vi "main.vi"() -> ()   [LabVIEW 2019]
uses:
  Type defs/Loop data Type Def.ctl
  Type defs/Persistent Type Def.ctl
  Type defs/Temp handle Type Def.ctl
  Type defs/Temp ctrl Type Def.ctl
  Custom devices/Custom temp ctrl settings.ctl
  Type defs/Paths Type Def.ctl
  Type defs/Settings Type Def.ctl
  Type defs/Imps Type Def.ctl
  Type defs/Source-meter Type Def.ctl
  Custom devices/Custom source-meter settings.ctl
  Type defs/Other settings Type Def.ctl
  Type defs/IV properties Type Def.ctl
  Type defs/CV properties Type Def.ctl
  Type defs/DLTS properties Type Def.ctl
  Type defs/LDLTS properties Type Def.ctl
  Type defs/MFIA handle Type Def.ctl
  <instrlib>/Zurich Instruments LabOne/Public/ziTypeHandle.ctl
  <instrlib>/Zurich Instruments LabOne/Public/Modules/ziTypeModHandle.ctl
  Type defs/Source-meter handle Type Def.ctl
  <vilib>/Utility/sysdir.llb/System Directory Type.ctl
  <vilib>/Utility/miscctls.llb/LVPointTypeDef.ctl
  <vilib>/Utility/error.llb/DialogType.ctl
  <instrlib>/Zurich Instruments LabOne/Zurich Instruments LabOne.lvlib
panel:
  out "Version":dbl caption="Numeric" format="myDLTS %.;%.2g"
  in  "Help":bool
  in  "Settings":bool
  in  "Path":path
  in  "File Open":bool
  in  "Add":bool
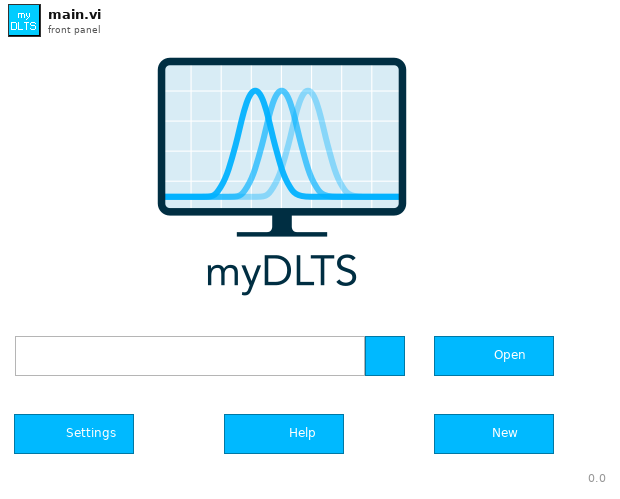
[diagram p1: front panel]
types:
  T1 = enum32{"Invalid", "Standard", "Closed", "Hidden", "Minimized", "Maximized"}
  T2 = typedef "System Directory Type.ctl" = i32
  T3 = typedef "LVPointTypeDef.ctl" = cluster{"Horizontal":i16, "Vertical":i16}
  T4 = typedef "Loop data Type Def.ctl" = cluster{"Persistent":T5, "Temp handle":T6, "Paths":T9, "Settings":T10, "Software version":dbl, "MFIA handle":T19, "Source-meter handle":T22}
  T5 = typedef "Persistent Type Def.ctl" = cluster{"Last file":path, "Last user":string, "Users":cluster{"User":string, "Authors directory":path}[]}
  T6 = typedef "Temp handle Type Def.ctl" = cluster{"Connected":bool, "Temp ctrl":T7}
  T7 = typedef "Temp ctrl Type Def.ctl" = cluster{"Gain (P)":dbl, "Reset (I)":dbl, "Rate (D)":dbl, "Stabilization rate":dbl, "Stabilization delta":dbl, "Type":enum16{"Custom", "Lake Shore 325", "Lake Shore 331", "Lake Shore 332", "Lake Shore 335"}, "Custom temp ctrl":T8, "Lakeshore 325":cluster{"VISA name":refnum<visa-resource-name>, "Loop":u16, "Heater Range":u16, "Heater Resistance":u16, "Sample sensor":u16, "Fast sensor":u16, "Slow sensor":u16}, "Lakeshore 331":cluster{"VISA name":refnum<visa-resource-name>, "Loop":u16, "Heater Range":u16, "Sample sensor":u16, "Fast sensor":u16, "Slow sensor":u16}, "Lakeshore 332":cluster{"VISA name":refnum<visa-resource-name>, "Loop":u16, "Heater Range":u16, "Sample sensor":u16, "Fast sensor":u16, "Slow sensor":u16}, "Lakeshore 335":cluster{"VISA name":refnum<visa-resource-name>, "Loop":u16, "Sample sensor":u16, "Fast sensor":u16, "Slow sensor":u16, "Heater Range":u16, "Output mode":enum16{"Off", "Closed Loop PID", "Zone", "Open Loop", "Monitor Out", "Warmup Supply"}}}
  T8 = typedef "Custom temp ctrl settings.ctl" = cluster{"VISA resource name":refnum<visa-resource-name>}
  T9 = typedef "Paths Type Def.ctl" = cluster{"Manual":path, "Settings":path, "Persistent":path, "Work dir.":path}
  T10 = typedef "Settings Type Def.ctl" = cluster{"MFIA":T11, "Temp ctrl":T7, "Source-meter":T12, "Other":T14, "Defaults":cluster{"IV properties":T15, "CV properties":T16, "DLTS properties":T17, "LDLTS properties":T18}}
  T11 = typedef "Imps Type Def.ctl" = cluster{"Address":string, "Use compensation":bool, "Shut down gracefully":bool}
  T12 = typedef "Source-meter Type Def.ctl" = cluster{"Type":enum16{"Custom", "Keithley 2600"}, "Custom source-meter":T13, "Keithley 2600":cluster{"VISA name":refnum<visa-resource-name>}}
  T13 = typedef "Custom source-meter settings.ctl" = cluster{"VISA resource name":refnum<visa-resource-name>}
  T14 = typedef "Other settings Type Def.ctl" = cluster{"Enable OriginLab":bool, "Reader mode":bool, "Auto-save":bool}
  T15 = typedef "IV properties Type Def.ctl" = cluster{"T":dbl[unit], "Vstart":dbl[unit], "Vstop":dbl[unit], "Vpoints":dbl, "Settling":dbl[unit], "I limit":dbl[unit], "Log mapping":bool, "Averaging":dbl}
  T16 = typedef "CV properties Type Def.ctl" = cluster{"T":dbl[unit], "Vstart":dbl[unit], "Vstop":dbl[unit], "Vpoints":dbl, "Precision":enum16{"Low (Fast)", "Normal", "High (Slow)"}, "Test signal":dbl[unit], "Auto I range":bool, "Test frequency":dbl[unit], "I range":dbl, "V range":dbl[unit], "Log mapping":bool, "Rel perm":dbl, "Area":dbl[unit]}
  T17 = typedef "DLTS properties Type Def.ctl" = cluster{"Tstart":dbl[unit], "Instant start":bool, "Tstop":dbl[unit], "T rate":dbl[unit], "Test signal":dbl[unit], "Test frequency":dbl[unit], "Bandwidth":dbl[unit], "Averaging":dbl, "Vbias":dbl[unit], "Vpulse":dbl[unit], "pulse length":dbl[unit], "Pulse 2":bool, "Vpulse 2":dbl[unit], "pulse length 2":dbl[unit], "I range":dbl, "V range":dbl[unit], "Emission rate":dbl[unit][], "Sampling rate":dbl[unit], "Acq. delay":dbl[unit]}
  T18 = typedef "LDLTS properties Type Def.ctl" = cluster{"T":dbl[unit], "Test signal":dbl[unit], "Test frequency":dbl[unit], "Bandwidth":dbl[unit], "Averaging":dbl, "Vbias":dbl[unit], "Vpulse":dbl[unit], "pulse length":dbl[unit], "Pulse 2":bool, "Vpulse 2":dbl[unit], "pulse length 2":dbl[unit], "I range":dbl, "V range":dbl[unit], "Sampling rate":dbl[unit], "Acq. delay":dbl[unit], "Sampling time":dbl[unit]}
  T19 = typedef "MFIA handle Type Def.ctl" = cluster{"ziHandle":T20, "Selected device":string, "ziModHandle":T21}
  T20 = typedef "Zurich Instruments LabOne.lvlib/ziTypeHandle.ctl" = cluster{"handleValid":bool, "Conn":u64, "Path Prefix":string, "Handle":u64, "Connected":bool, "Clockbase(s)":dbl}
  T21 = typedef "Zurich Instruments LabOne.lvlib/ziTypeModHandle.ctl" = cluster{"handleValid":bool, "Conn":u64, "ModHandle":u64, "moduleID":string, "Path Prefix":string}
  T22 = typedef "Source-meter handle Type Def.ctl" = cluster{"Connected":bool, "Source-meter":T12}
  T23 = enum8{"Enabled", "Disabled", "Disabled and Grayed Out"}
  T24 = typedef "DialogType.ctl" = u16
  T25 = typedef "Session properties Type Def.ctl" = cluster{"Session name":string, "Comment":string, "User":string, "Software version":dbl, "Created":timestamp, "Modified":timestamp, "Binary":bool, "GUID":string}
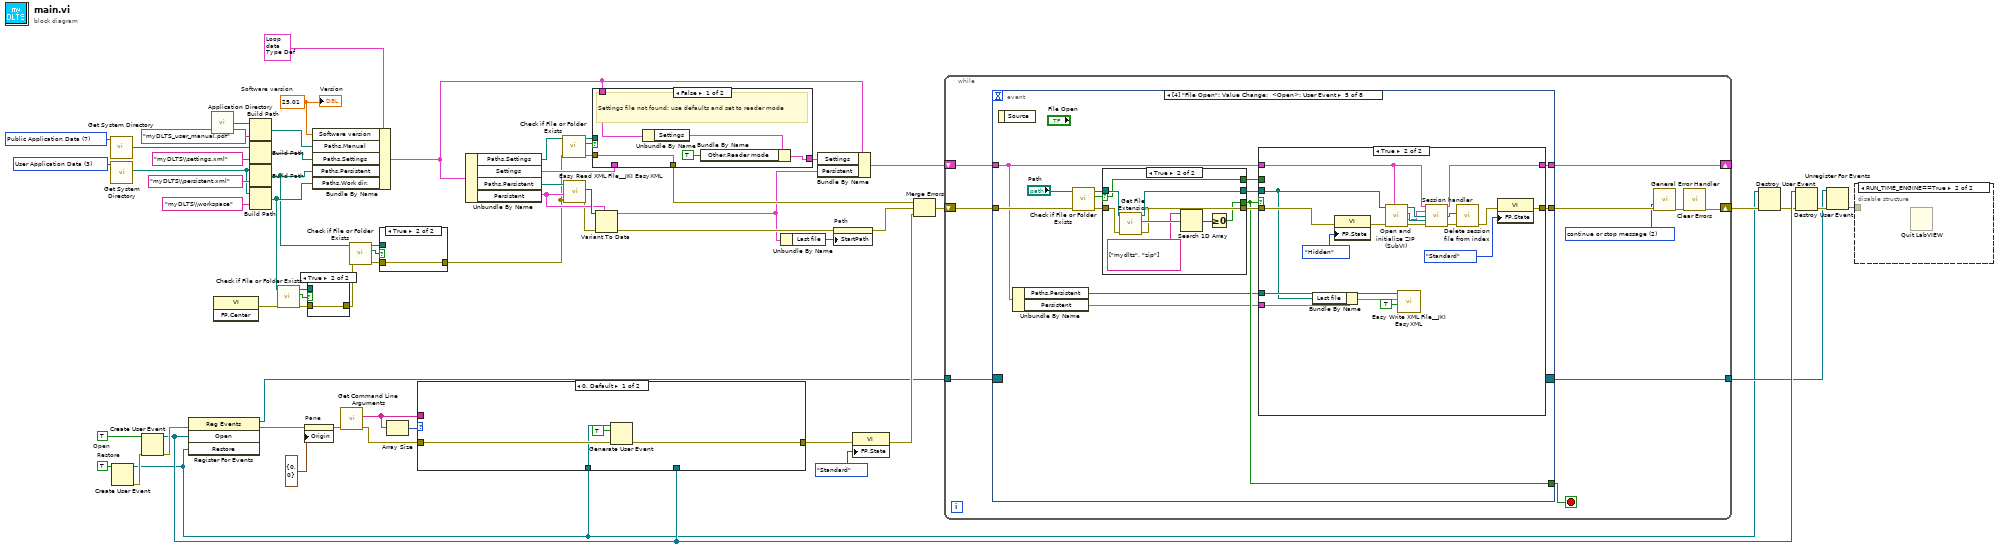
[diagram p0: block diagram]
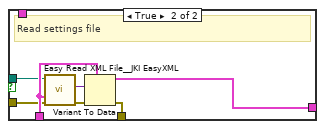
[diagram p2: hidden frame]
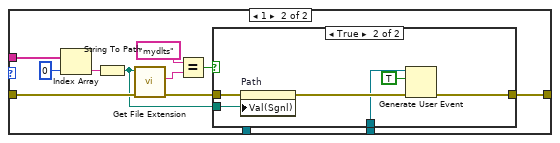
[diagram p4: hidden frame]
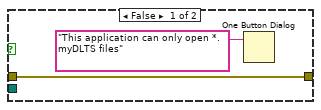
[diagram p5: hidden frame]
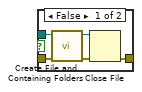
[diagram p6: hidden frame]
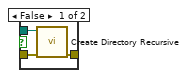
[diagram p7: hidden frame]
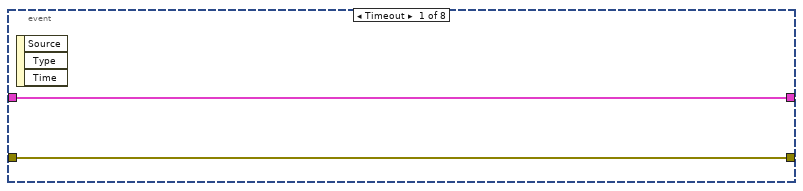
[diagram p8: hidden frame]
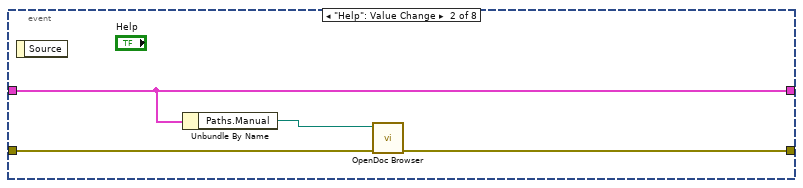
[diagram p9: hidden frame]
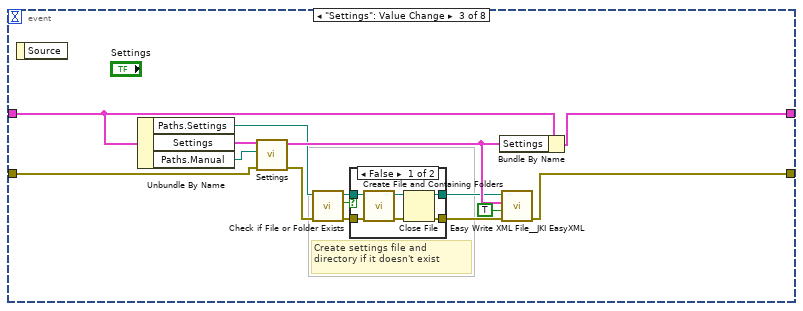
[diagram p10: hidden frame]
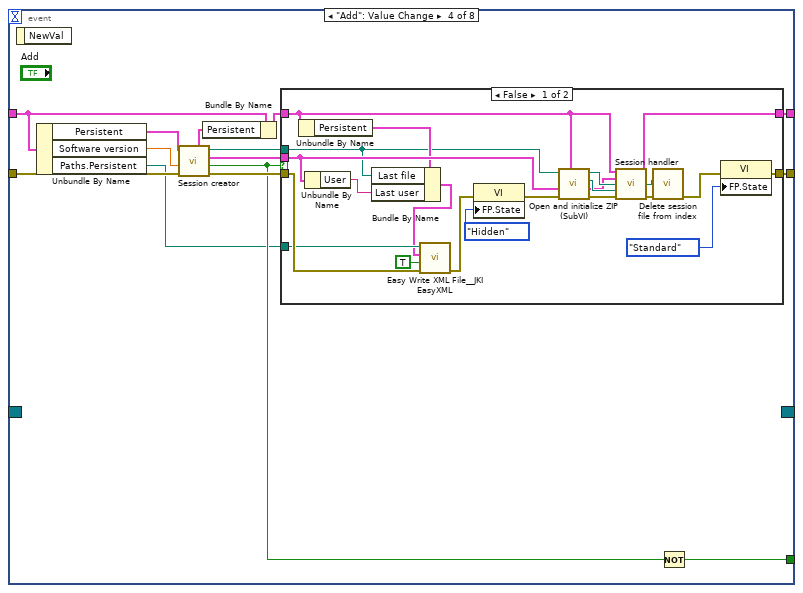
[diagram p12: hidden frame]
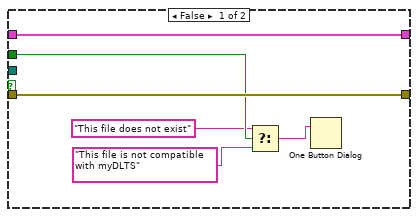
[diagram p15: hidden frame]
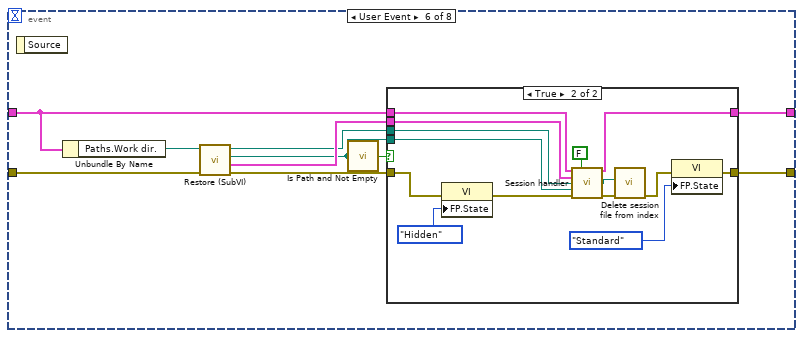
[diagram p16: hidden frame]
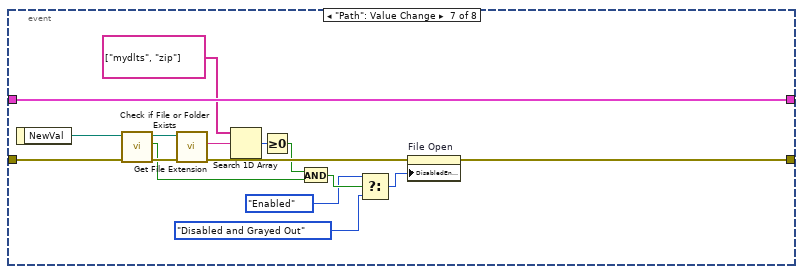
[diagram p18: hidden frame]
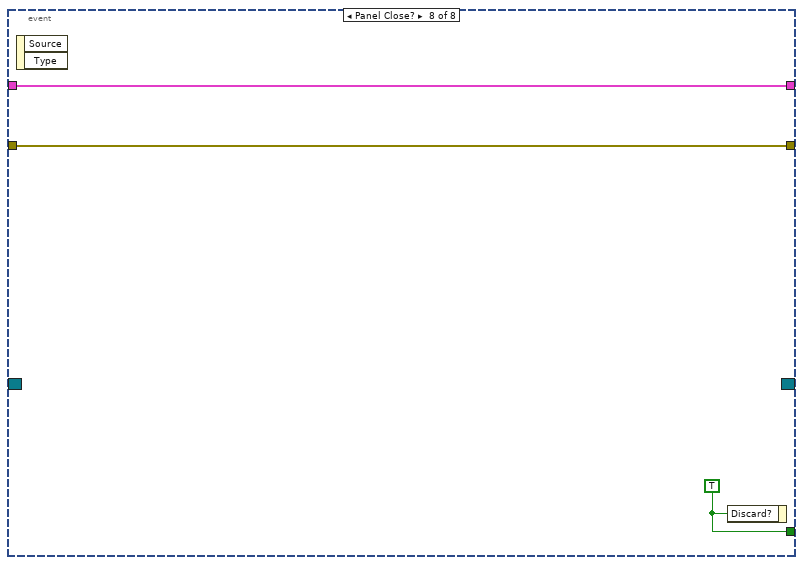
[diagram p19: hidden frame]
diagram:
  w1 = 25.01  # Software version
  w12 = TRUE  # Restore
  w20 = TRUE  # Open
  w30 = T2 7 items=["User Home"=0, "User Desktop"=1, "User Documents"=2, "User Application Data"=3, "User Preferences"=4, "User Temporary"=5, "Public Documents"=6, "Public Application Data"=7, "Public Preferences"=8, "Public Cache"=13, "System Core Libraries"=9, "System Installed Libraries"=10, "Application Files"=11, "Boot Volume Root"=12] ("system directory type")
  w59 = T2 3 items=["User Home"=0, "User Desktop"=1, "User Documents"=2, "User Application Data"=3, "User Preferences"=4, "User Temporary"=5, "Public Documents"=6, "Public Application Data"=7, "Public Preferences"=8, "Public Cache"=13, "System Core Libraries"=9, "System Installed Libraries"=10, "Application Files"=11, "Boot Volume Root"=12] ("system directory type")
  n1 = call <vilib>:"Get System Directory.vi"("system directory type"=w30) -> ("system directory"=w29:path)  [unwired: 10 in]
  n2 = call <vilib>:"Get System Directory.vi"("system directory type"=w59) -> ("system directory"=w56:path)  [unwired: 10 in]
  n3 = Create User Event(user event datatype=w12) -> (user event=w8:refnum<user-event>, error out=w11:errorcluster)  [unwired: 1 in]
  n4 = Create User Event(user event datatype=w20, error in=w11) -> (user event=w16:refnum<user-event>, error out=w17:errorcluster)
  n5 = register-events(error in=w17, w16, w8) -> (reference out=w18:refnum<event-registration>, error out=w19:errorcluster)  [unwired: 1 in]
  n6 = call <vilib>:"Application Directory.vi"() -> ("Application Directory"=w62:path)
  n7 = invoke class="VI" method="FP.Center"() -> (error out=w21:errorcluster)  [unwired: 3 in, 2 out]
  n8 = Build Path(base path=w62, name or relative path="myDLTS_user_manual.pdf") -> (appended path=w60:path)
  n9 = Build Path(base path=w29, name or relative path="myDLTS\\settings.xml") -> (appended path=w36:path)
  n10 = Build Path(base path=w56, name or relative path="myDLTS\\persistent.xml") -> (appended path=w38:path)
  n11 = Build Path(base path=w56, name or relative path="myDLTS\\workspace") -> (appended path=w45:path)
  n12 = call <vilib>:"Check if File or Folder Exists.vi"("error in (no error)"=w21, "path"=w45) -> ("error out"=w43:errorcluster, "file or folder exists?"=w42:bool, "dup path"=w44:path)  [unwired: 7 in]
  n13 = property on="Pane" class="Pane"(error in=w19, "Origin"=T3 {"Horizontal"=0, "Vertical"=0}) -> (error out=w32:errorcluster)  [unwired: 1 in, 1 out]
  n14 = case shown="True" w42 {
    tunnel: w44 -> [w66 _]
    tunnel: w43 -> [w65 w67]
    tunnel: [w64 w67] -> w37
    frame False {
      n15 = call <vilib>:"Create Directory Recursive.vi"("error in (no error)"=w65, "directory"=w66) -> ("error out"=w64:errorcluster)  [unwired: 3 in, 2 out]
    }
    frame True {
    }
  }
  n16 = Bundle By Name(cluster=T4 {"Persistent"={"Last file"=path "", "Last user"="", "Users"=[]}, "Temp handle"={"Connected"=FALSE, "Temp ctrl"={"Gain (P)"=0.0, "Reset (I)"=0.0, "Rate (D)"=0.0, "Stabilization rate"=0.0, "Stabilization delta"=0.0, "Type"=enum."Lake Shore 325", "Custom temp ctrl"={"VISA resource name"=""}, "Lakeshore 325"={"VISA name"="", "Loop"=0, "Heater Range"=1, "Heater Resistance"=0, "Sample sensor"=0, "Fast sensor"=0, "Slow sensor"=0}, "Lakeshore 331"={"VISA name"="", "Loop"=1, "Heater Range"=0, "Sample sensor"=0, "Fast sensor"=0, "Slow sensor"=0}, "Lakeshore 332"={"VISA name"="", "Loop"=1, "Heater Range"=0, "Sample sensor"=0, "Fast sensor"=0, "Slow sensor"=0}, "Lakeshore 335"={"VISA name"="", "Loop"=1, "Sample sensor"=0, "Fast sensor"=0, "Slow sensor"=0, "Heater Range"=0, "Output mode"=enum."Off"}}}, "Paths"={"Manual"=path "", "Settings"=path "", "Persistent"=path "", "Work dir."=path ""}, "Settings"={"MFIA"={"Address"="", "Use compensation"=FALSE, "Shut down gracefully"=FALSE}, "Temp ctrl"={"Gain (P)"=0.0, "Reset (I)"=0.0, "Rate (D)"=0.0, "Stabilization rate"=0.1, "Stabilization delta"=0.5, "Type"=enum."Custom", "Custom temp ctrl"={"VISA resource name"=""}, "Lakeshore 325"={"VISA name"="", "Loop"=1, "Heater Range"=1, "Heater Resistance"=1, "Sample sensor"=0, "Fast sensor"=0, "Slow sensor"=0}, "Lakeshore 331"={"VISA name"="", "Loop"=1, "Heater Range"=0, "Sample sensor"=0, "Fast sensor"=0, "Slow sensor"=0}, "Lakeshore 332"={"VISA name"="", "Loop"=1, "Heater Range"=0, "Sample sensor"=0, "Fast sensor"=0, "Slow sensor"=0}, "Lakeshore 335"={"VISA name"="", "Loop"=1, "Sample sensor"=0, "Fast sensor"=0, "Slow sensor"=0, "Heater Range"=0, "Output mode"=enum."Off"}}, "Source-meter"={"Type"=enum."Custom", "Custom source-meter"={"VISA resource name"=""}, "Keithley 2600"={"VISA name"=""}}, "Other"={"Enable OriginLab"=FALSE, "Reader mode"=FALSE, "Auto-save"=FALSE}, "Defaults"={"IV properties"={"T"=300.0, "Vstart"=-3.0, "Vstop"=3.0, "Vpoints"=101.0, "Settling"=0.0, "I limit"=0.001, "Log mapping"=FALSE, "Averaging"=10.0}, "CV properties"={"T"=300.0, "Vstart"=-10.0, "Vstop"=0.0, "Vpoints"=101.0, "Precision"=enum."Normal", "Test signal"=0.1, "Auto I range"=TRUE, "Test frequency"=1000000.0, "I range"=-2.0, "V range"=10.0, "Log mapping"=FALSE, "Rel perm"=0.0, "Area"=0.0}, "DLTS properties"={"Tstart"=200.0, "Instant start"=FALSE, "Tstop"=300.0, "T rate"=0.016666666666666666, "Test signal"=0.1, "Test frequency"=1000000.0, "Bandwidth"=5000.0, "Averaging"=10.0, "Vbias"=-4.0, "Vpulse"=0.0, "pulse length"=0.001, "Pulse 2"=FALSE, "Vpulse 2"=0.0, "pulse length 2"=0.001, "I range"=-2.0, "V range"=10.0, "Emission rate"=[10.0, 20.0, 50.0, 100.0, 200.0, 500.0, 1000.0], "Sampling rate"=107142.859375, "Acq. delay"=0.0}, "LDLTS properties"={"T"=300.0, "Test signal"=0.1, "Test frequency"=1000000.0, "Bandwidth"=5000.0, "Averaging"=100.0, "Vbias"=-4.0, "Vpulse"=0.0, "pulse length"=0.001, "Pulse 2"=FALSE, "Vpulse 2"=0.0, "pulse length 2"=0.001, "I range"=-2.0, "V range"=10.0, "Sampling rate"=107142.859375, "Acq. delay"=0.0, "Sampling time"=1.25}}}, "Software version"=0.0, "MFIA handle"={"ziHandle"={"handleValid"=FALSE, "Conn"=0, "Path Prefix"="", "Handle"=0, "Connected"=FALSE, "Clockbase(s)"=0.0}, "Selected device"="", "ziModHandle"={"handleValid"=FALSE, "Conn"=0, "ModHandle"=0, "moduleID"="", "Path Prefix"=""}}, "Source-meter handle"={"Connected"=FALSE, "Source-meter"={"Type"=enum."Keithley 2600", "Custom source-meter"={"VISA resource name"=""}, "Keithley 2600"={"VISA name"=""}}}}, "Software version"=w1, "Paths.Manual"=w60, "Paths.Settings"=w36, "Paths.Persistent"=w38, "Paths.Work dir."=w45) -> (w3:T4)
  n17 = call <vilib>:"Get Command Line Arguments.vi"("error in (no error)"=w32) -> ("error out"=w33:errorcluster, "arguments"=w34:string[])  [unwired: 8 in, 1 out]
  n18 = call <vilib>:"Check if File or Folder Exists.vi"("error in (no error)"=w37, "path"=w38) -> ("error out"=w40:errorcluster, "file or folder exists?"=w39:bool, "dup path"=w41:path)  [unwired: 7 in]
  n19 = case shown="True" w39 {
    tunnel: w41 -> [w70 _]
    tunnel: w40 -> [w69 w73]
    tunnel: [w68 w73] -> w2
    frame False {
      n20 = call <vilib>:"Create File and Containing Folders.vi"("error in (no error)"=w69, "file path"=w70) -> ("error out"=w71:errorcluster, "refnum out"=w72:refnum<file>)  [unwired: 8 in]
      n21 = Close File(refnum=w72, error in=w71) -> (error out=w68:errorcluster)  [unwired: 1 out]
    }
    frame True {
    }
  }
  n22 = Array Size(array=w34) -> (size(s)=w35:i32)
  n23 = case shown="0, Default" w35 {
    tunnel: w34 -> [_ w88]
    tunnel: w33 -> [w76 w86]
    tunnel: [w75 w80] -> w23
    tunnel: w16 -> [_ w78]
    tunnel: w8 -> [w74 _]
    frame 0, Default {
      n24 = Generate User Event(user event=w74, event data cluster=TRUE ("event data"), error in=w76) -> (error out=w75:errorcluster)  [unwired: 1 in, 1 out]
    }
    frame 1 {
      n25 = Index Array(array=w88, index=0) -> (element=w82:string)
      n26 = String To Path(string=w82) -> (path=w79:path)
      n27 = call <vilib>:"Get File Extension.vi"("error in (no error)"=w86, "file"=w79) -> ("error out"=w81:errorcluster, "lowercase file extension"=w85:string)  [unwired: 5 in, 3 out]
      n28 = Equal?(x="mydlts", y=w85) -> (x = y?=w83:bool)
      n29 = case shown="True" w83 {
        tunnel: w79 -> [_ w95]
        tunnel: w81 -> [w90 w96]
        tunnel: [w90 w93] -> w80
        tunnel: w78 -> [_ w92]
        frame False {
          n30 = One Button Dialog(message="This application can only open *.myDLTS files") -> ()  [unwired: 1 in, 1 out]
        }
        frame True {
          n31 = property on="Path" class="Path"(error in=w96, "Val(Sgnl)"=w95) -> (error out=w94:errorcluster)  [unwired: 1 in, 1 out]
          n32 = Generate User Event(user event=w92, event data cluster=TRUE ("event data"), error in=w94) -> (error out=w93:errorcluster)  [unwired: 1 in, 1 out]
        }
      }
    }
  }
  n33 = Unbundle By Name(w3) -> ("Paths.Settings"=w6:path, "Settings"=w50:T10, "Paths.Persistent"=w54:path, "Persistent"=w52:T5)
  n34 = call <vilib>:"Check if File or Folder Exists.vi"("error in (no error)"=w2, "path"=w6) -> ("error out"=w7:errorcluster, "file or folder exists?"=w4:bool, "dup path"=w5:path)  [unwired: 7 in]
  n35 = call <vilib>:"Easy Read XML File__JKI EasyXML.vi"("error in (no error)"=w2, "LabVIEW Data (Type)"=w52, "XML File Path"=w54) -> ("error out"=w51:errorcluster, "LabVIEW Data"=w53:variant)  [unwired: 6 in, 1 out]
  n36 = case shown="False" w4 {
    tunnel: w50 -> [_ w106]
    tunnel: [w97 w105] -> w48
    tunnel: [w101 w104] -> w47
    tunnel: w7 -> [w101 w103]
    tunnel: w5 -> [_ w102]
    tunnel: w3 -> [w100 _]
    frame False {
      # "Settings file not found; use defaults and set to reader mode"
      n37 = Unbundle By Name(w100) -> ("Settings"=w99:T10)
      n38 = Bundle By Name(cluster=w99, "Other.Reader mode"=TRUE) -> (w97:T10)
    }
    frame True {
      # "Read settings file"
      n39 = call <vilib>:"Easy Read XML File__JKI EasyXML.vi"("error in (no error)"=w103, "LabVIEW Data (Type)"=w106, "XML File Path"=w102) -> ("error out"=w107:errorcluster, "LabVIEW Data"=w108:variant)  [unwired: 6 in, 1 out]
      n40 = Variant To Data(error in=w107, type=w106, Variant=w108) -> (data=w105:T10, error out=w104:errorcluster)
    }
  }
  n41 = Variant To Data(error in=w51, type=w52, Variant=w53) -> (data=w26:T5, error out=w28:errorcluster)
  n42 = Unbundle By Name(w26) -> ("Last file"=w25:path)
  n43 = Bundle By Name(cluster=w3, "Settings"=w48, "Persistent"=w26) -> (w49:T4)
  n44 = property on="Path" class="Path"(error in=w28, "StartPath"=w25) -> (error out=w27:errorcluster)  [unwired: 1 in, 1 out]
  n45 = property on="Property Node" class="VI"(error in=w23, "FP.State"=T1."Standard" ("Front Panel Window:State")) -> (error out=w22:errorcluster)  [unwired: 1 in, 1 out]
  n46 = Merge Errors(w47, w27, w22) -> (w46:errorcluster)
  n47 = while {
    shift-right: [w115] -> _
    shift-left: w49 -> [w117]
    shift-right: [w109] -> w10
    shift-left: w46 -> [w116]
    tunnel: w18 -> [w111]
    tunnel: [w110] -> w13
    stop <- w118 stop-if-true
    w112 = T24 2 items=["no dialog", "OK message", "continue or stop message", "OK message + warnings", "continue/stop + warnings"] ("type of dialog (OK msg:1)")
    n48 = event shown="[4] \"File Open\": Value Change;  <Open>: User Event" {
      selector: w111 -> [_ _ _ _ _ _ _ _]
      dyn-events: [_ _ _ _ _ _ _ _] -> w110
      timeout: _ -> [_ _ _ _ _ _ _ _]
      tunnel: [_ _ _ w153 w188 _ _ w281] -> w118
      tunnel: w117 -> [w120 w124 w137 w150 w197 w246 w278 w280]
      tunnel: w116 -> [w119 w123 w139 w161 w198 w242 w277 w279]
      tunnel: [w120 w124 w136 w158 w195 w244 w278 w280] -> w115
      tunnel: [w119 w122 w133 w157 w196 w245 w267 w279] -> w114
      event Timeout {
        n49 = event-data() -> ()  [unwired: 1 in, 3 out]
      }
      event "Help": Value Change {
        n50 = event-data() -> ()  [unwired: 1 in, 1 out]
        n51 = Unbundle By Name(w124) -> ("Paths.Manual"=w121:path)
        n52 = call "OpenDoc Browser.vi"("error in (no error)"=w123, "File"=w121) -> ("error out"=w122:errorcluster)  [unwired: 9 in]
      }
      event "Settings": Value Change {
        # "Create settings file and directory if it doesn't exist"
        n53 = event-data() -> ()  [unwired: 1 in, 1 out]
        n54 = Unbundle By Name(w137) -> ("Paths.Settings"=w127:path, "Settings"=w138:T10, "Paths.Manual"=w132:path)
        n55 = call "Settings.vi"("Error In"=w139, "Manual"=w132, "Settings in"=w138) -> ("Error Out"=w128:errorcluster, "Settings"=w135:T10)  [unwired: 7 in]
        n56 = call <vilib>:"Check if File or Folder Exists.vi"("error in (no error)"=w128, "path"=w127) -> ("error out"=w129:errorcluster, "file or folder exists?"=w131:bool, "dup path"=w130:path)  [unwired: 7 in]
        n57 = case shown="False" w131 {
          tunnel: w130 -> [w145 w147]
          tunnel: w129 -> [w144 w146]
          tunnel: [w141 w147] -> w125
          tunnel: [w140 w146] -> w126
          frame False {
            n58 = call <vilib>:"Create File and Containing Folders.vi"("error in (no error)"=w144, "file path"=w145) -> ("error out"=w143:errorcluster, "refnum out"=w142:refnum<file>)  [unwired: 8 in]
            n59 = Close File(refnum=w142, error in=w143) -> (path=w141:path, error out=w140:errorcluster)
          }
          frame True {
          }
        }
        n60 = Bundle By Name(cluster=w137, "Settings"=w135) -> (w136:T4)
        n61 = call <vilib>:"Easy Write XML File__JKI EasyXML.vi"("error in (no error)"=w126, "Overwrite File? (false)"=TRUE, "LabVIEW Data"=w135, "XML File Path"=w125) -> ("error out"=w133:errorcluster)  [unwired: 6 in, 1 out]
      }
      event "Add": Value Change {
        n62 = event-data() -> ()  [unwired: 1 in, 1 out]
        n63 = Unbundle By Name(w150) -> ("Persistent"=w151:T5, "Software version"=w156:dbl, "Paths.Persistent"=w152:path)
        n64 = call "Session creator.vi"("error in (no error)"=w161, "Software version"=w156, "Persistent In"=w151) -> ("error out"=w155:errorcluster, "Canceled"=w154:bool, "Session properties"=w160:T25, "Created file"=w159:path, "Persistent Out"=w149:T5)  [unwired: 4 in]
        n65 = Bundle By Name(cluster=w150, "Persistent"=w149) -> (w148:T4)
        n66 = case shown="False" w154 {
          tunnel: w155 -> [w171 w184]
          tunnel: w160 -> [w168 _]
          tunnel: w159 -> [w165 _]
          tunnel: w148 -> [w167 w185]
          tunnel: [w175 w185] -> w158
          tunnel: [w181 w184] -> w157
          tunnel: w152 -> [w169 _]
          frame False {
            n67 = Unbundle By Name(w167) -> ("Persistent"=w166:T5)
            n68 = Unbundle By Name(w168) -> ("User"=w164:string)
            n69 = Bundle By Name(cluster=w166, "Last file"=w165, "Last user"=w164) -> (w163:T5)
            n70 = call <vilib>:"Easy Write XML File__JKI EasyXML.vi"("error in (no error)"=w171, "Overwrite File? (false)"=TRUE, "LabVIEW Data"=w163, "XML File Path"=w169) -> ("error out"=w170:errorcluster)  [unwired: 6 in, 1 out]
            n71 = property on="Property Node" class="VI"(error in=w170, "FP.State"=T1."Hidden" ("Front Panel Window:State")) -> (error out=w177:errorcluster)  [unwired: 1 in, 1 out]
            n72 = call "Open and initialize ZIP (SubVI).vi"("Loop Data"=w167, "error in (no error)"=w177, "Session properties"=w168, "File to be opened"=w165) -> ("error out"=w180:errorcluster, "Session properties out"=w176:T25, "Opened file"=w178:path, "Workspace target"=w179:path)  [unwired: 4 in]
            n73 = call "Session handler.vi"("Loop data"=w167, "Session properties"=w176, "Workspace base"=w179, "Actual file"=w178, "Error In"=w180) -> ("Loop data out"=w175:T4, "Workspace out"=w174:path, "Error Out"=w173:errorcluster)  [unwired: 5 in, 3 out]
            n74 = call "Delete session file from index.vi"("Workspace path"=w174, "error in (no error)"=w173) -> ("error out"=w172:errorcluster)  [unwired: 7 in, 1 out]
            n75 = property on="Property Node" class="VI"(error in=w172, "FP.State"=T1."Standard" ("Front Panel Window:State")) -> (error out=w181:errorcluster)  [unwired: 1 in, 1 out]
          }
          frame True {
          }
        }
        n76 = Not(x=w154) -> (.not. x?=w153:bool)
      }
      event "File Open": Value Change; User Event {
        n77 = event-data() -> ()  [unwired: 1 in, 1 out]
        n78 = Unbundle By Name(w197) -> ("Paths.Persistent"=w187:path, "Persistent"=w186:T5)
        n79 = call <vilib>:"Check if File or Folder Exists.vi"("error in (no error)"=w198, "path"="Path") -> ("error out"=w193:errorcluster, "file or folder exists?"=w194:bool, "dup path"=w192:path)  [unwired: 7 in]
        n80 = case shown="True" w194 {
          selector: w194 -> [w200 w203]
          tunnel: w193 -> [w201 w210]
          tunnel: w192 -> [w202 w209]
          tunnel: [w202 w207] -> w191
          tunnel: [w201 w208] -> w190
          tunnel: [w200 w204] -> w188
          tunnel: [w200 w203] -> w189
          frame False {
          }
          frame True {
            n81 = call <vilib>:"Get File Extension.vi"("error in (no error)"=w210, "file"=w209) -> ("error out"=w208:errorcluster, "lowercase file extension"=w211:string, "dup file"=w207:path)  [unwired: 5 in, 2 out]
            n82 = Search 1D Array(1D array=string[] ["mydlts", "zip"], element=w211) -> (index of element=w205:i32)  [unwired: 1 in]
            n83 = Greater Or Equal To 0?(x=w205) -> (x >= 0?=w204:bool)
          }
        }
        n84 = case shown="True" w188 {
          tunnel: w190 -> [w216 w234]
          tunnel: w191 -> [_ w219]
          tunnel: w197 -> [w217 w223]
          tunnel: [w217 w227] -> w195
          tunnel: [w216 w233] -> w196
          tunnel: w189 -> [w215 _]
          tunnel: w187 -> [_ w222]
          tunnel: w186 -> [_ w221]
          frame False {
            n85 = Select(t="This file does not exist" ("f"), s=w215, f="This file is not compatible with myDLTS") -> (s? t:f=w214:string)
            n86 = One Button Dialog(message=w214) -> ()  [unwired: 1 in, 1 out]
          }
          frame True {
            n87 = Bundle By Name(cluster=w221, "Last file"=w219) -> (w220:T5)
            n88 = property on="Property Node" class="VI"(error in=w234, "FP.State"=T1."Hidden" ("Front Panel Window:State")) -> (error out=w229:errorcluster)  [unwired: 1 in, 1 out]
            n89 = call "Open and initialize ZIP (SubVI).vi"("Loop Data"=w223, "error in (no error)"=w229, "File to be opened"=w219) -> ("error out"=w232:errorcluster, "Session properties out"=w228:T25, "Opened file"=w230:path, "Workspace target"=w231:path)  [unwired: 5 in]
            n90 = call <vilib>:"Easy Write XML File__JKI EasyXML.vi"("Overwrite File? (false)"=TRUE, "LabVIEW Data"=w220, "XML File Path"=w222) -> ()  [unwired: 7 in, 2 out]
            n91 = call "Session handler.vi"("Loop data"=w223, "Session properties"=w228, "Workspace base"=w231, "Actual file"=w230, "Error In"=w232) -> ("Loop data out"=w227:T4, "Workspace out"=w226:path, "Error Out"=w225:errorcluster)  [unwired: 5 in, 3 out]
            n92 = call "Delete session file from index.vi"("Workspace path"=w226, "error in (no error)"=w225) -> ("error out"=w224:errorcluster)  [unwired: 7 in, 1 out]
            n93 = property on="Property Node" class="VI"(error in=w224, "FP.State"=T1."Standard" ("Front Panel Window:State")) -> (error out=w233:errorcluster)  [unwired: 1 in, 1 out]
          }
        }
      }
      event User Event {
        n94 = event-data() -> ()  [unwired: 1 in, 1 out]
        n95 = Unbundle By Name(w246) -> ("Paths.Work dir."=w243:path)
        n96 = call "Restore (SubVI).vi"("error in (no error)"=w242, "Workspace"=w243) -> ("error out"=w241:errorcluster, "Session properties"=w240:T25, "ZIP file path"=w237:path, "Workspace path"=w239:path)  [unwired: 5 in, 1 out]
        n97 = call <vilib>:"Is Path and Not Empty.vi"("path"=w237) -> ("Is Path and Not Empty?"=w238:bool)  [unwired: 4 in]
        n98 = case shown="True" w238 {
          tunnel: w241 -> [w247 w260]
          tunnel: w246 -> [w248 w254]
          tunnel: [w248 w258] -> w244
          tunnel: [w247 w259] -> w245
          tunnel: w240 -> [_ w253]
          tunnel: w239 -> [_ w252]
          tunnel: w237 -> [_ w251]
          frame False {
          }
          frame True {
            n99 = property on="Property Node" class="VI"(error in=w260, "FP.State"=T1."Hidden" ("Front Panel Window:State")) -> (error out=w250:errorcluster)  [unwired: 1 in, 1 out]
            n100 = call "Session handler.vi"("Loop data"=w254, "Has been propperly saved?"=FALSE, "Session properties"=w253, "Workspace base"=w252, "Actual file"=w251, "Error In"=w250) -> ("Loop data out"=w258:T4, "Workspace out"=w257:path, "Error Out"=w256:errorcluster)  [unwired: 4 in, 3 out]
            n101 = call "Delete session file from index.vi"("Workspace path"=w257, "error in (no error)"=w256) -> ("error out"=w255:errorcluster)  [unwired: 7 in, 1 out]
            n102 = property on="Property Node" class="VI"(error in=w255, "FP.State"=T1."Standard" ("Front Panel Window:State")) -> (error out=w259:errorcluster)  [unwired: 1 in, 1 out]
          }
        }
      }
      event "Path": Value Change {
        n103 = event-data() -> ("NewVal"=w275:path)  [unwired: 1 in]
        n104 = call <vilib>:"Check if File or Folder Exists.vi"("error in (no error)"=w277, "path"=w275) -> ("error out"=w276:errorcluster, "file or folder exists?"=w272:bool, "dup path"=w274:path)  [unwired: 7 in]
        n105 = call <vilib>:"Get File Extension.vi"("error in (no error)"=w276, "file"=w274) -> ("error out"=w273:errorcluster, "lowercase file extension"=w264:string)  [unwired: 5 in, 3 out]
        n106 = Search 1D Array(1D array=string[] ["mydlts", "zip"], element=w264) -> (index of element=w266:i32)  [unwired: 1 in]
        n107 = Greater Or Equal To 0?(x=w266) -> (x >= 0?=w263:bool)
        n108 = And(x=w263, y=w272) -> (x .and. y?=w271:bool)
        n109 = Select(t=T23."Enabled" ("Disabled"), s=w271, f=T23."Disabled and Grayed Out") -> (s? t:f=w269:T23)
        n110 = property on="File Open" class="Bool"(error in=w273, "DisabledEnum"=w269) -> (error out=w267:errorcluster)  [unwired: 1 in, 1 out]
      }
      event Panel Close? {
        w281 = TRUE
        n111 = event-data() -> ()  [unwired: 1 in, 2 out]
        n112 = event-data("Discard?"=w281) -> ()  [unwired: 1 in, 1 out]
      }
    }
    n113 = call <vilib>:"General Error Handler.vi"("type of dialog (OK msg:1)"=w112, "error in (no error)"=w114) -> ("error out"=w113:errorcluster)  [unwired: 9 in, 4 out]
    n114 = call <vilib>:"Clear Errors.vi"("error in (no error)"=w113) -> ("error out"=w109:errorcluster)  [unwired: 5 in, 1 out]
  }
  n115 = Destroy User Event(user event=w8, error in=w10) -> (error out=w9:errorcluster)
  n116 = Destroy User Event(user event=w16, error in=w9) -> (error out=w15:errorcluster)
  n117 = Unregister For Events(event registration refnum=w13, error in=w15) -> (error out=w14:errorcluster)
  n118 = disable-structure shown="RUN_TIME_ENGINE==True" {
    disable-tunnel: w14 -> [_ _]
    frame condition #0 (active) {
    }
    frame condition #1 {
      n119 = Quit LabVIEW() -> ()  [unwired: 1 in]
    }
  }
  "Version" <- w1
